vi "TDMS Delete Retry.vi"(8 "error in":errorcluster, 9 "confirm (F)":bool, 10 "entire hierarchy (F)":bool, 11 "path (use dialog)":path) -> (0 "error out":errorcluster, 3 "deleted path":path)   [LabVIEW 2011]
uses:
  Summitek EXT/OpenG EXT/file/file.llb/File Exists - Scalar__ogtk.vi
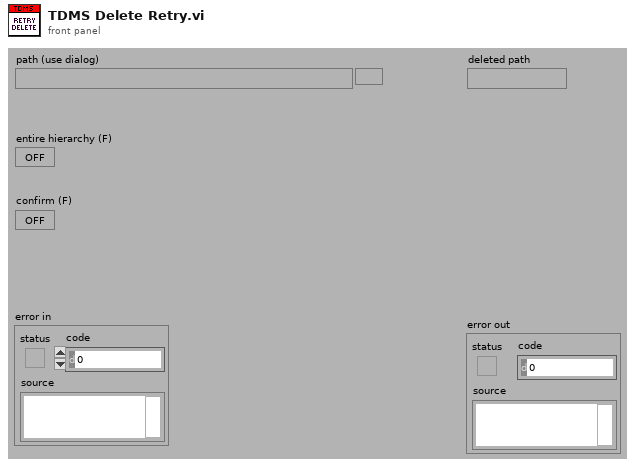
[diagram p1: front panel]
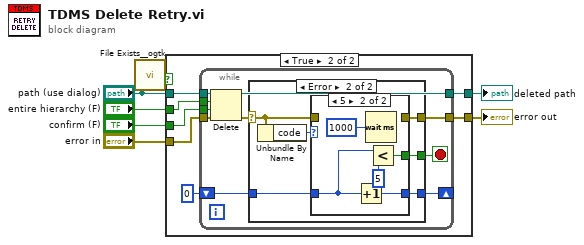
[diagram p0: block diagram]
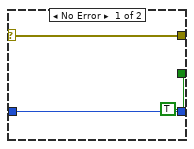
[diagram p3: hidden frame]
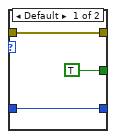
[diagram p4: hidden frame]
diagram:
  n1 = call-poly "File Exists__ogtk.vi"("file path"="path (use dialog)") -> ("exists"=w1:bool)  [unwired: 6 in, 1 out]
  n2 = case shown="True" w1 {
    tunnel: "path (use dialog)" -> [w8 w16]
    tunnel: [w9 w15] -> w7
    tunnel: "entire hierarchy (F)" -> [_ w14]
    tunnel: "confirm (F)" -> [_ w13]
    tunnel: "error in" -> [w9 w12]
    tunnel: [w8 w11] -> w3
    frame False {
      # "Don't try to delete if the\nfile does not exist."
    }
    frame True {
      n3 = while {
        tunnel: w16 -> [w26]
        tunnel: [w20] -> w15
        tunnel: w14 -> [w25]
        tunnel: w13 -> [w24]
        tunnel: w12 -> [w23]
        tunnel: [w22] -> w11
        shift-right: [w17] -> _
        shift-left: 0 -> [w18]
        stop <- w19 stop-if-true
        n4 = Delete(path (use dialog)=w26, entire hierarchy (F)=w25, confirm (F)=w24, error in=w23) -> (deleted path=w22:path, error out=w21:errorcluster)  [unwired: 2 out]
        n5 = case shown="Error" w21 {
          selector: w21 -> [w29 w33]
          tunnel: [w29 w30] -> w20
          tunnel: [TRUE w34] -> w19
          tunnel: w18 -> [w27 w32]
          tunnel: [w27 w31] -> w17
          frame No Error {
          }
          frame Error {
            n6 = Unbundle By Name(w33) -> ("code"=w35:i32)
            n7 = case shown="5" w35 {
              tunnel: [TRUE w42] -> w34
              tunnel: w33 -> [w36 _]
              tunnel: w32 -> [w37 w40]
              tunnel: [w37 w39] -> w31
              tunnel: [w36 _] -> w30
              frame Default {
              }
              frame 5 {
                n8 = Increment(x=w40) -> (x+1=w39:i32)
                n9 = Wait (ms)(milliseconds to wait=u32 1000) -> ()  [unwired: 1 out]
                n10 = Less?(x=w40, y=5 ("milliseconds to wait")) -> (x < y?=w42:bool)
              }
            }
          }
        }
      }
    }
  }
  "error out" <- w7
  "deleted path" <- w3
